vi "Corridor to Diag. Scale.vi"(8 "Command Info In":T2, 10 "Corridor to Diag Scale":T1={"Target Angle"=38.0, "Distance"=55.0, "Speed"=0.65, "Scale Height"=6.0}, 11 "Starting Position":T5) -> (0 "Command Info Out":T2)   [LabVIEW 2017]
uses:
  <vilib>/Rock Robotics/WPI/Framework/Command Status Info.ctl
  <vilib>/Rock Robotics/WPI/Framework/Completion Status.ctl
  <vilib>/Rock Robotics/WPI/Framework/Completion Notifier.ctl
  Support Code/Starting Position.ctl
  Block Clusters/Corridor to Diag Scale.ctl
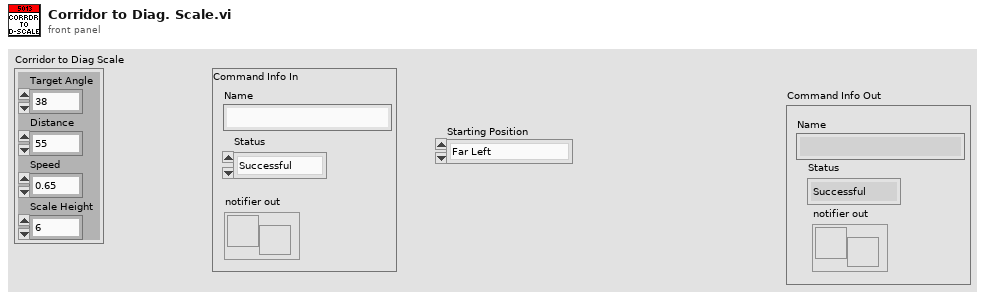
[diagram p1: front panel]
types:
  T1 = typedef "Corridor to Diag Scale.ctl" = cluster{"Target Angle":dbl, "Distance":dbl, "Speed":dbl, "Scale Height":dbl}
  T2 = typedef "Command Status Info.ctl" = cluster{"Name":string, "Status":T3, "notifier out":T4}
  T3 = typedef "Completion Status.ctl" = enum16{"Successful", "Aborted", "Incomplete"}
  T4 = typedef "Completion Notifier.ctl" = refnum<notifier>
  T5 = typedef "Starting Position.ctl" = enum16{"Far Left", "Center", "Far Right"}
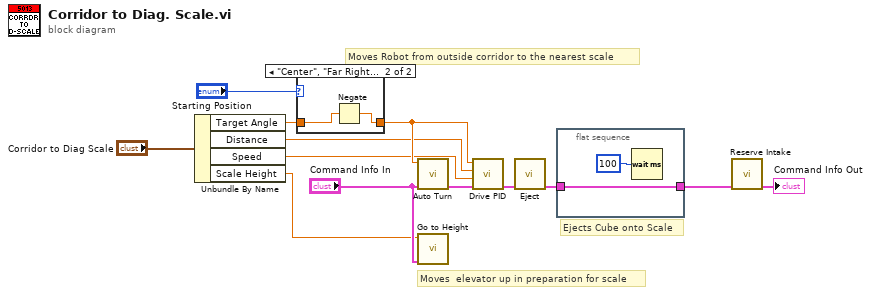
[diagram p0: block diagram]
diagram:
  # "Ejects Cube onto Scale"
  # "Moves  elevator up in preparation for scale"
  # "Moves Robot from outside corridor to the nearest scale"
  n1 = Unbundle By Name("Corridor to Diag Scale") -> ("Target Angle"=w4:dbl, "Distance"=w3:dbl, "Speed"=w2:dbl, "Scale Height"=w1:dbl)
  n2 = case shown="\"Center\", \"Far Right\"" "Starting Position" {
    tunnel: [w14 w16] -> w12
    tunnel: w4 -> [w14 w15]
    frame "Far Left", Default {
    }
    frame "Center", "Far Right" {
      n3 = Negate(x=w15) -> (-x=w16:dbl)
    }
  }
  n4 = call "Auto Turn.vi"("Command Info In"="Command Info In", "Target Angle"=w12) -> ("Command Info Out"=w11:T2)  [unwired: 9 in]
  n5 = call "Go to Height.vi"("Command Info In"="Command Info In", "Target Height (in)"=w1) -> ()  [unwired: 9 in, 1 out]
  n6 = call "Drive PID.vi"("Command Info In"=w11, "Speed"=w2, "Distance"=w3, "Target Angle"=w12) -> ("Command Info Out"=w9:T2)  [unwired: 7 in]
  n7 = call "Eject.vi"("Command Info In"=w9) -> ("Command Info Out"=w8:T2)  [unwired: 10 in]
  n8 = flat-sequence {
    tunnel: w8 -> [w17]
    tunnel: [w17] -> w6
    frame #0 {
      n9 = Wait (ms)(milliseconds to wait=u32 100) -> ()  [unwired: 1 out]
    }
  }
  n10 = call "Reserve Intake.vi"("Command Info"=w6) -> ("Command Info"=→"Command Info Out":T2)  [unwired: 10 in]
